vi "Configure Calibration Kit.vi"(7 "Connector type":T1(ring), 8 "error in (no error)":errorcluster, 10 "Cal kit Name":string, 11 "VNA-CMT S2 S4 in":refnum<class "VNA-CMT S2 S4.lvclass">) -> (0 "error out":errorcluster, 3 "VNA-CMT S2 S4 out":refnum<class "VNA-CMT S2 S4.lvclass">)   [LabVIEW 2020, in "VNA-CMT S2 S4.lvclass"]
doc: "Configure the calibration kit to use."
uses:
  VNA-CMT S2 S4.lvclass
  Vector Network Analyzer.lvclass
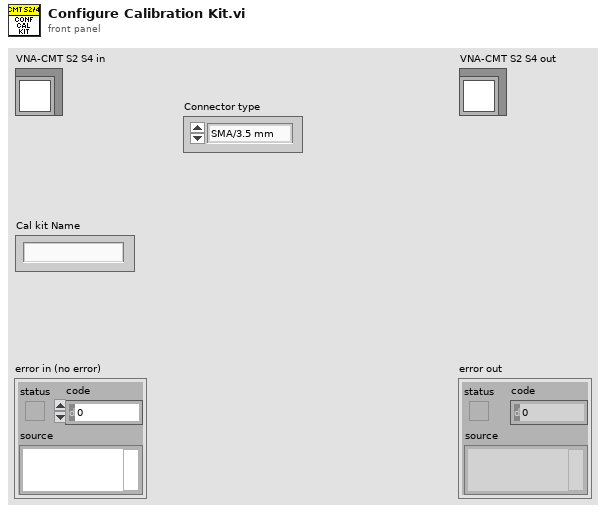
[diagram p1: front panel]
types:
  T1 = enum16{"SMA/3.5 mm", "2.92 mm", "2.4 mm", "1.85 mm", "N 50 Ohm", "N 75 Ohm", "7-16"}
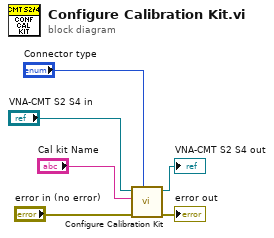
[diagram p0: block diagram]
diagram:
  n1 = call-parent "Configure Calibration Kit.vi"("Connector type"="Connector type", "error in (no error)"="error in (no error)", "Cal kit Name"="Cal kit Name", "Vector Network Analyzer in"="VNA-CMT S2 S4 in") -> ("error out"=→"error out":errorcluster, "Vector Network Analyzer out"=→"VNA-CMT S2 S4 out":refnum<class "VNA-CMT S2 S4.lvclass">)  [unwired: 6 in]
